vi "PYBD2_Code.vi"() -> ()   [LabVIEW 2020]
uses:
  Subs/ColorText/Code.xctl
  Subs/Console XCtrl/Console_Xctrl.xctl
panel:
  in  "Clean":bool
  in  "Tree":string(tree)
  in  "PC Save":bool
  in  "New File":bool
  in  "Base Path":path
  in  "Code":string(xcontrol)="import os\n\nfor i in range(10):\n     print(i)\n"
  in  "Files":bool
  in  "Stop":bool
  in  "Run":bool
  out "REPL":string(xcontrol)
  in  "Help files":u16(ring) items=["BlinkLED.py", "BreathingLED.py", "DAQ_12bit.py", "DAQ_8bit.py", "Debounce.py", "InLineAssembly.py", "interrupts.py", "MotorController.py", "neopixels.py", "Screen.py", "Servo.py", "SImpleUART.py", "Stepper.py", "Switch_callback.py", "SystemLink.py", "Tacho_interrupts.py", "Tacho_loop.py", "TempTile.py", "Timers_callbacks.py", "UART_Passthrough.py", "WiFi.py"]
  out "Help Code":string(xcontrol)="import os\n\nfor i in range(10):\n     print(i)\n"
  # "PyBoard"
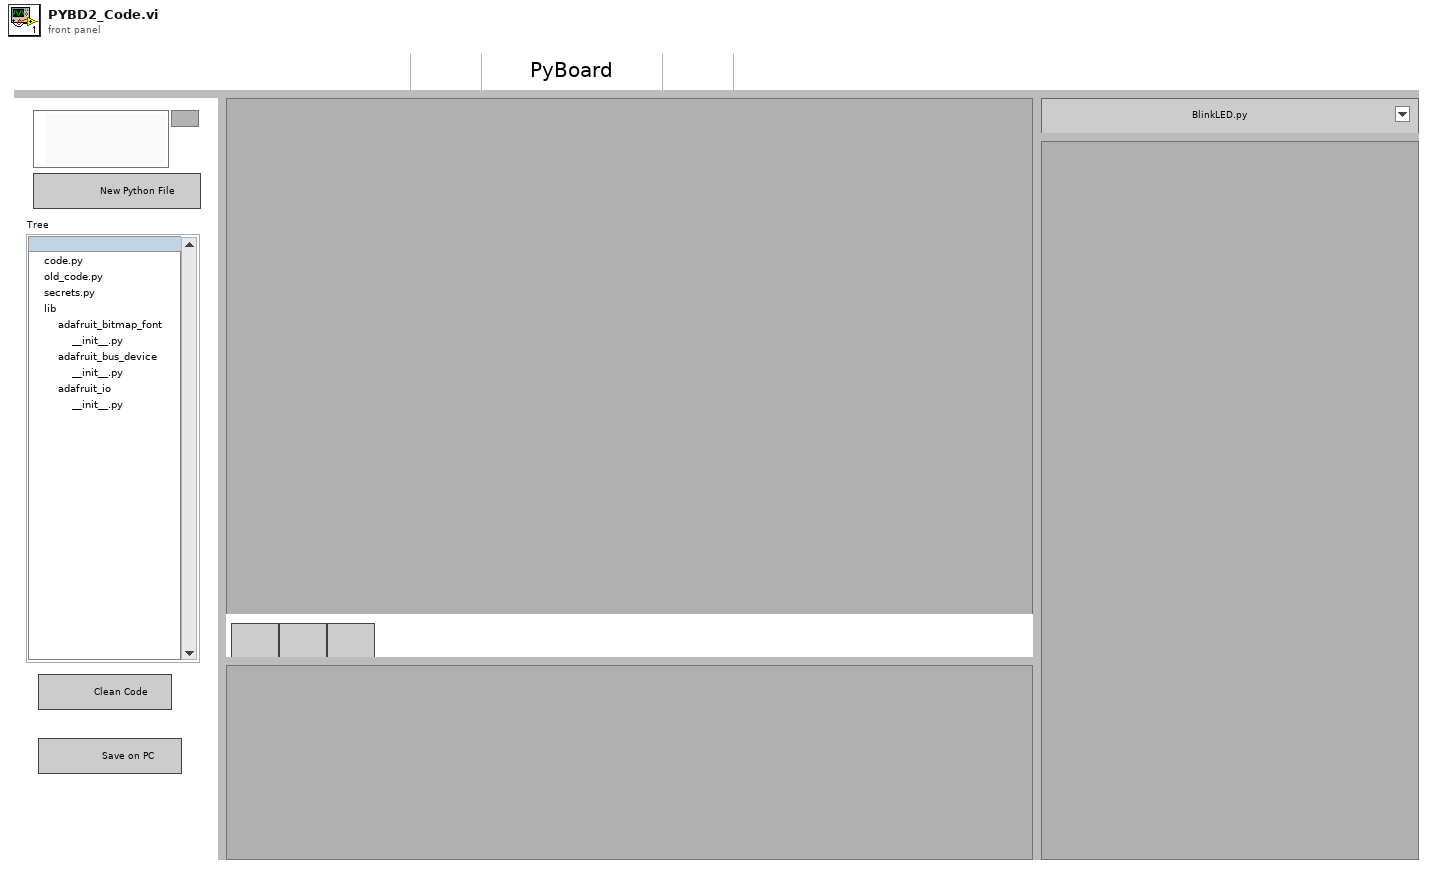
[diagram p1: front panel]
types:
  T1 = cluster{"Quote":u32, "Comment":u32, "Python":u32, "Text":u32, "Triple Quote":u32, "function":u32, "Line numbers":u32, "REPL Err":u32, "REPL Text":u32, "Text Bkgd":u32, "REPL Bkgd":u32}
  T2 = typedef "eventvkey.ctl" = enum16{"ASCII", "Enter", "Return", "Shift", "Ctrl", "Alt", "Cmd", "Opt", "Caps", "NumLock", "Clear", "Break", "Up", "Down", "Left", "Right", "Insert", "Delete", "Home", "End", "PageUp", "PageDown", "Escape", "Help", "Pause", "ScrollLock", "F1", "F2", "F3", "F4", "F5", "F6", "F7", "F8", "F9", "F10", "F11", "F12", "F13", "F14", "F15", "F16", "F17", "F18", "F19", "F20", "F21", "F22", "F23", "F24", "Play", "VolumeUp", "VolumeDown", "Mute", "Two Byte Char"}
  T3 = cluster{"Shift":bool, "Ctrl":bool, "Alt":bool, "Cmd":bool, "Opt":bool}
  T4 = cluster{"Char":i16, "VKey":T2, "PlatMods":cluster{"Shift":bool, "Ctrl":bool, "Alt":bool, "Cmd":bool, "Opt":bool}}
  T5 = enum8{"Enabled", "Disabled", "Disabled and Grayed Out"}
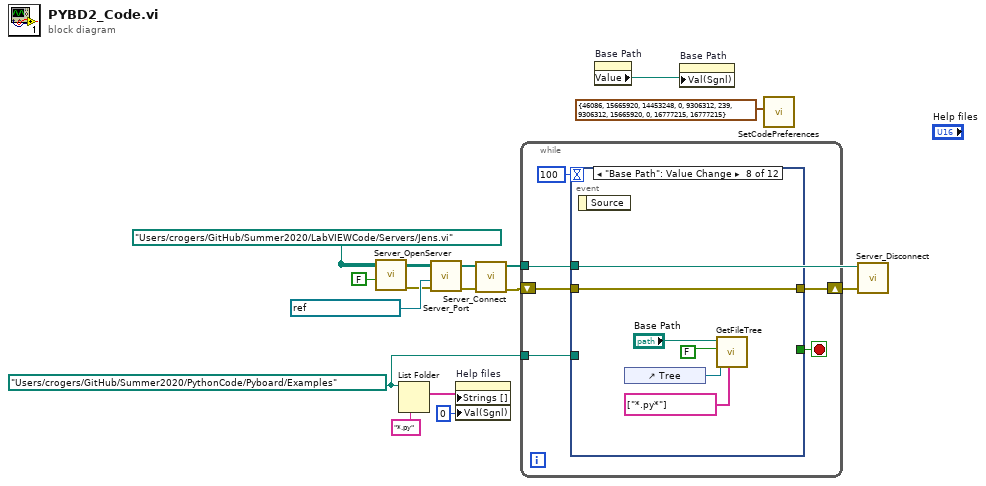
[diagram p0: block diagram]
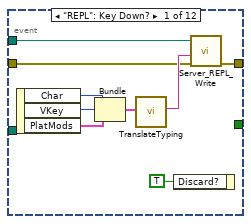
[diagram p2: hidden frame]
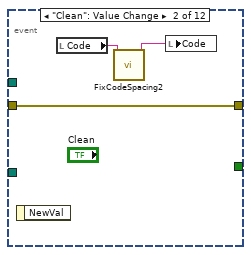
[diagram p3: hidden frame]
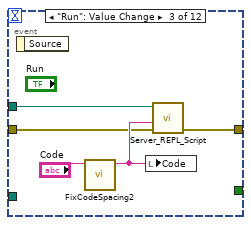
[diagram p4: hidden frame]
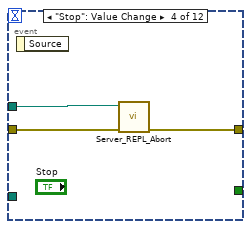
[diagram p5: hidden frame]
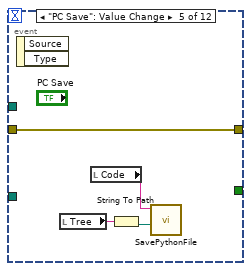
[diagram p6: hidden frame]
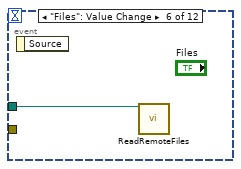
[diagram p7: hidden frame]
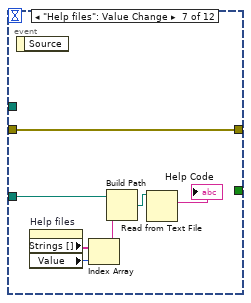
[diagram p8: hidden frame]
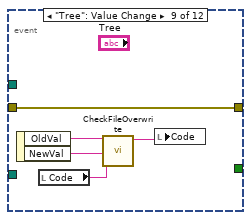
[diagram p9: hidden frame]
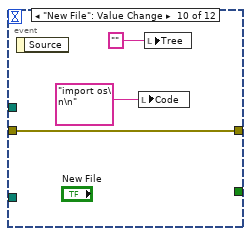
[diagram p10: hidden frame]
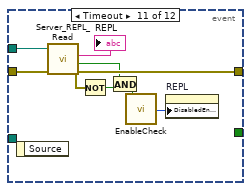
[diagram p11: hidden frame]
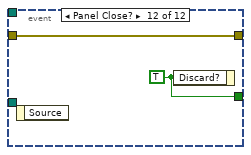
[diagram p12: hidden frame]
diagram:
  w3 = path "/Users/crogers/GitHub/Summer2020/PythonCode/Pyboard/Examples"
  w7 = path "/Users/crogers/GitHub/Summer2020/LabVIEWCode/Servers/Jens.vi" ("Server")
  n1 = call "Server_OpenServer.vi"("Wait for connection?"=FALSE, "Server"=w7) -> ("error out"=w11:errorcluster)  [unwired: 9 in]
  n2 = List Folder(path=w3, pattern="*.py") -> (filenames=w5:string[])  [unwired: 2 in, 3 out]
  n3 = call "Server_Port.vi"("error in (no error)"=w11, "Port"=refnum<visa-resource-name> "ASRL22::INSTR", "Server"=w7) -> ("error out"=w10:errorcluster)  [unwired: 8 in]
  n4 = property on="Help files" class="Ring (strict)"("Strings []"=w5, "Val(Sgnl)"=0) -> ()  [unwired: 2 in, 2 out]
  n5 = call "Server_Connect.vi"("error in (no error)"=w10, "Server"=w7) -> ("error out"=w9:errorcluster)  [unwired: 9 in]
  n6 = while {
    tunnel: w7 -> [w17]
    shift-right: [w18] -> w8
    shift-left: w9 -> [w19]
    tunnel: w3 -> [w14]
    stop <- w15 stop-if-true
    n7 = event shown="[7] \"Base Path\": Value Change" {
      selector: _ -> [_ _ _ _ _ _ _ _ _ _ _ _]
      dyn-events: _ -> [_ _ _ _ _ _ _ _ _ _ _ _]
      timeout: 100 -> [_ _ _ _ _ _ _ _ _ _ _ _]
      tunnel: w19 -> [w25 w31 w34 w39 w40 _ w45 w56 w61 w64 w71 w73]
      tunnel: [w24 w31 w33 w38 w40 _ w45 w56 w61 w64 w67 w73] -> w18
      tunnel: w17 -> [w20 _ w32 w37 _ w44 _ _ _ _ w72 _]
      tunnel: [_ _ _ _ _ _ _ _ _ _ _ w74] -> w15
      tunnel: w14 -> [_ _ _ _ _ _ w49 _ _ _ _ _]
      event "REPL": Key Down? {
        n8 = event-data() -> ("Char"=w22:i16, "VKey"=w23:T2, "PlatMods"=w21:T3)  [unwired: 1 in]
        n9 = Bundle("Char"=w22, "VKey"=w23, "PlatMods"=w21) -> (w27:T4)  [unwired: 1 in]
        n10 = call "TranslateTyping.vi"("Cluster"=w27) -> ("key"=w28:string)  [unwired: 10 in]
        n11 = event-data("Discard?"=TRUE) -> ()  [unwired: 1 in, 1 out]
        n12 = call "Server_REPL_Write.vi"("error in (no error)"=w25, "Code"=w28, "Server"=w20) -> ("error out"=w24:errorcluster)  [unwired: 8 in]
      }
      event "Clean": Value Change {
        n13 = event-data() -> ()  [unwired: 1 in, 1 out]
        n14 = local read "Code"() -> (w30:string)
        n15 = call "FixCodeSpacing2.vi"("Code"=w30) -> ("Cleaned"=w29:string)  [unwired: 10 in]
        n16 = local write "Code"(w29) -> ()
      }
      event "Run": Value Change {
        n17 = event-data() -> ()  [unwired: 1 in, 1 out]
        n18 = call "FixCodeSpacing2.vi"("Code"="Code") -> ("Cleaned"=w36:string)  [unwired: 10 in]
        n19 = local write "Code"(w36) -> ()
        n20 = call "Server_REPL_Script.vi"("error in (no error)"=w34, "Code"=w36, "Server"=w32) -> ("error out"=w33:errorcluster)  [unwired: 8 in]
      }
      event "Stop": Value Change {
        n21 = event-data() -> ()  [unwired: 1 in, 1 out]
        n22 = call "Server_REPL_Abort.vi"("error in (no error)"=w39, "Server"=w37) -> ("error out"=w38:errorcluster)  [unwired: 9 in]
      }
      event "PC Save": Value Change {
        n23 = event-data() -> ()  [unwired: 1 in, 2 out]
        n24 = local read "Tree"() -> (w41:string)
        n25 = local read "Code"() -> (w42:string)
        n26 = String To Path(string=w41) -> (path=w43:path)
        n27 = call "SavePythonFile.vi"("path"=w43, "Code"=w42) -> ()  [unwired: 10 in]
      }
      event "Files": Value Change {
        n28 = event-data() -> ()  [unwired: 1 in, 1 out]
        n29 = call "ReadRemoteFiles.vi"("Server"=w44) -> ()  [unwired: 11 in]
      }
      event "Help files": Value Change {
        n30 = event-data() -> ()  [unwired: 1 in, 1 out]
        n31 = property on="Help files" class="Ring (strict)"() -> ("Strings []"=w51:string[], "Value"=w50:u16)  [unwired: 2 in, 2 out]
        n32 = Index Array(array=w51, index=w50) -> (element=w48:string)
        n33 = Build Path(base path=w49, name or relative path=w48) -> (appended path=w47:path)
        n34 = Read from Text File(file (use dialog)=w47) -> (text=→"Help Code":string)  [unwired: 3 in, 3 out]
      }
      event "Base Path": Value Change {
        n35 = event-data() -> ()  [unwired: 1 in, 1 out]
        n36 = control-ref of="Tree"() -> (w54:refnum<vi>)
        n37 = call "GetFileTree.vi"("patterns"=string[] ["*.py*"], "Tree"=w54, "Open?"=FALSE, "Base Path"="Base Path") -> ()  [unwired: 8 in]
      }
      event "Tree": Value Change {
        n38 = event-data() -> ("OldVal"=w60:string, "NewVal"=w59:string)  [unwired: 1 in]
        n39 = local read "Code"() -> (w57:string)
        n40 = call "CheckFileOverwrite.vi"("Current Code"=w57, "New Value"=w59, "Old Value"=w60) -> ("Code out"=w58:string)  [unwired: 8 in]
        n41 = local write "Code"(w58) -> ()
      }
      event "New File": Value Change {
        n42 = event-data() -> ()  [unwired: 1 in, 1 out]
        n43 = local write "Code"("import os\n\n") -> ()
        n44 = local write "Tree"("") -> ()
      }
      event Timeout {
        n45 = event-data() -> ()  [unwired: 1 in, 1 out]
        n46 = call "Server_REPL_Read.vi"("error in (no error)"=w71, "Server"=w72) -> ("error out"=w67:errorcluster, "Running?"=w66:bool, "REPL"=→"REPL":string)  [unwired: 7 in]
        n47 = Not(x=w67) -> (.not. x?=w68:bool)
        n48 = And(x=w66, y=w68) -> (x .and. y?=w65:bool)
        n49 = call "EnableCheck.vi"("Enable?"=w65) -> ("Enum"=w69:T5)
        n50 = property on="REPL" class="Console_Xctrl (strict)"("DisabledEnum"=w69) -> ()  [unwired: 2 in, 2 out]
      }
      event Panel Close? {
        w74 = TRUE ("Discard?")
        n51 = event-data() -> ()  [unwired: 1 in, 1 out]
        n52 = event-data("Discard?"=w74) -> ()  [unwired: 1 in, 1 out]
      }
    }
  }
  n53 = property on="Base Path" class="Path"() -> ("Value"=w2:path)  [unwired: 2 in, 2 out]
  n54 = property on="Base Path" class="Path"("Val(Sgnl)"=w2) -> ()  [unwired: 2 in, 2 out]
  n55 = call "SetCodePreferences.vi"("Color choices"=T1 {"Quote"=46086, "Comment"=15665920, "Python"=14453248, "Text"=0, "Triple Quote"=9306312, "function"=239, "Line numbers"=9306312, "REPL Err"=15665920, "REPL Text"=0, "Text Bkgd"=16777215, "REPL Bkgd"=16777215}) -> ()  [unwired: 11 in]
  n56 = call "Server_Disconnect.vi"("error in (no error)"=w8, "Server"=w7) -> ()  [unwired: 9 in, 1 out]
